vi "testFailureMessageWithVI.vi"() -> ()   [LabVIEW 2019, in "AssertionTest.lvlib" / "AssertNotRefnum.lvlib"]
uses:
  AssertNotRefnum.lvlib
  Assertion/Assertion.lvlib
panel:
  out "error out":errorcluster
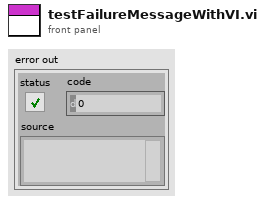
[diagram p1: front panel]
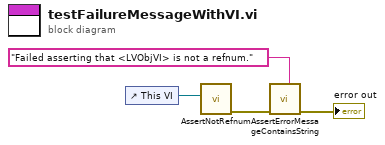
[diagram p0: block diagram]
diagram:
  n1 = control-ref of="This VI"() -> (w2:refnum<vi>)
  n2 = call "AssertNotRefnum.vi"("Refnum"=w2) -> ("error out"=w4:errorcluster)  [unwired: 10 in]
  n3 = call "AssertErrorMessageContainsString.vi"("Expected"="Failed asserting that <LVObjVI> is not a refnum.", "error in (no error)"=w4) -> ("error out"=→"error out":errorcluster)  [unwired: 9 in]
